vi "TDS Waveform Output Clear.vi"(8 "error in (no error)":errorcluster, 10 "Signal InstConfig":string, 11 "Address":string) -> (0 "error out":errorcluster)   [LabVIEW 2025, in "Interface Functions.lvlib"]
uses:
  Interface Functions.lvlib
panel:
  # "Waveform Output Clear"
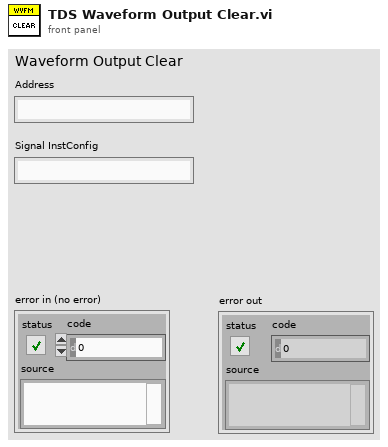
[diagram p1: front panel]
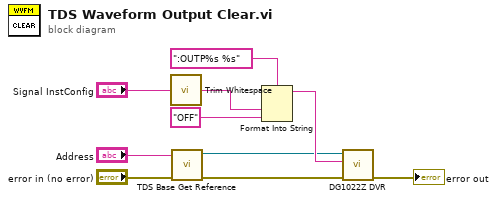
[diagram p0: block diagram]
diagram:
  n1 = call <vilib>:"Trim Whitespace.vi"("string"="Signal InstConfig") -> ("trimmed string"=w5:string)  [unwired: 1 in]
  n2 = call "TDS Base Get Reference.vi"("error in (no error)"="error in (no error)", "Address"="Address") -> ("error out"=w2:errorcluster, "Reference"=w3:refnum<visa-resource-name>)  [unwired: 8 in]
  n3 = Format Into String(format string=":OUTP%s %s", w5, "OFF") -> (resulting string=w4:string)  [unwired: 2 in, 1 out]
  n4 = call "DG1022Z DVR.vi"("error in (no error)"=w2, "write buffer"=w4, "VISA resource name"=w3) -> ("error out"=→"error out":errorcluster)  [unwired: 7 in, 1 out]
